vi "Write Limit Current.vi"(8 "error in":errorcluster, 10 "OverCurrent_Protect":dbl, 11 "69X_79X in":refnum<class "69X_79X.lvclass">) -> (0 "error out":errorcluster, 3 "69X_79X out":refnum<class "69X_79X.lvclass">)   [LabVIEW 2019, in "69X_79X.lvlib" / "69X_79X.lvclass"]
uses:
  Library/69X_79X.lvclass
  builds/Instruments/PowerSupply.lvlibp/Library/PowerSupply.lvclass
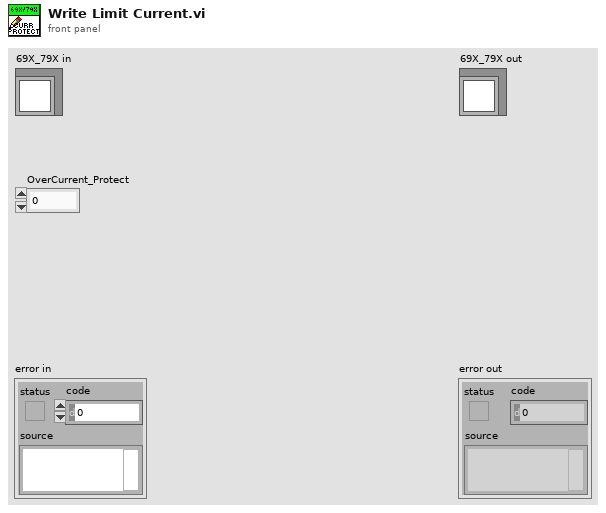
[diagram p1: front panel]
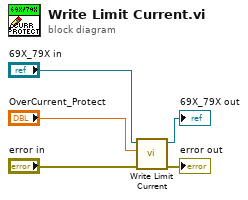
[diagram p0: block diagram]
diagram:
  n1 = call-parent "Write Limit Current.vi"("error in"="error in", "OverCurrent_Protect"="OverCurrent_Protect", "PowerSupply in"="69X_79X in") -> ("error out"=→"error out":errorcluster, "PowerSupply out"=→"69X_79X out":refnum<class "69X_79X.lvclass">)  [unwired: 7 in]
